vi "AuMT8852B EDR Relative Transmit Power Results.vi"(8 "error in (no error)":errorcluster, 11 "VISA session":refnum<visa-resource-name>) -> (0 "error out":errorcluster, 2 "error code":i32, 3 "VISA session out":refnum<visa-resource-name>, 4 "Results":T1 {"Peak 2DHx DPSK Absolute Power (dBm)" format="%.2f"; "Avg 2DHx DPSK Absolute Power (dBm)" format="%.2f"; "Min 2DHx DPSK Absolute Power (dBm)" format="%.2f"; "Max 2DHx DPSK Absolute Power (dBm)" format="%.2f"; "Peak 2DHx GFSK Absolute Power (dBm)" format="%.2f"; "Avg 2DHx GFSK Absolute Power (dBm)" format="%.2f"; "Min 2DHx GFSK Absolute Power (dBm)" format="%.2f"; "Max 2DHx GFSK Absolute Power (dBm)" format="%.2f"; "Peak 3DHx DPSK Absolute Power (dBm)" format="%.2f"; "Avg 3DHx DPSK Absolute Power (dBm)" format="%.2f"; "Min 3DHx DPSK Absolute Power (dBm)" format="%.2f"; "Max 3DHx DPSK Absolute Power (dBm)" format="%.2f"; "Peak 3DHx GFSK Absolute Power (dBm)" format="%.2f"; "Avg 3DHx GFSK Absolute Power (dBm)" format="%.2f"; "Min 3DHx GFSK Absolute Power (dBm)" format="%.2f"; "Max 3DHx GFSK Absolute Power (dBm)" format="%.2f"; "Avg power difference (dBm)" format="%.2f"; "Min power difference (dBm)" format="%.2f"; "Max power difference (dBm)" format="%.2f"; "Avg power difference (dBm)" format="%.2f"; "Min power difference (dBm)" format="%.2f"; "Max power difference (dBm)" format="%.2f"})   [LabVIEW 2017]
doc: "Anritsu MT8852B Bluetooth Tester\n\nReturns the summary results of the EDR Relative Transmit Power test.\n\nOUTPUT\nResults - measurements made during the test."
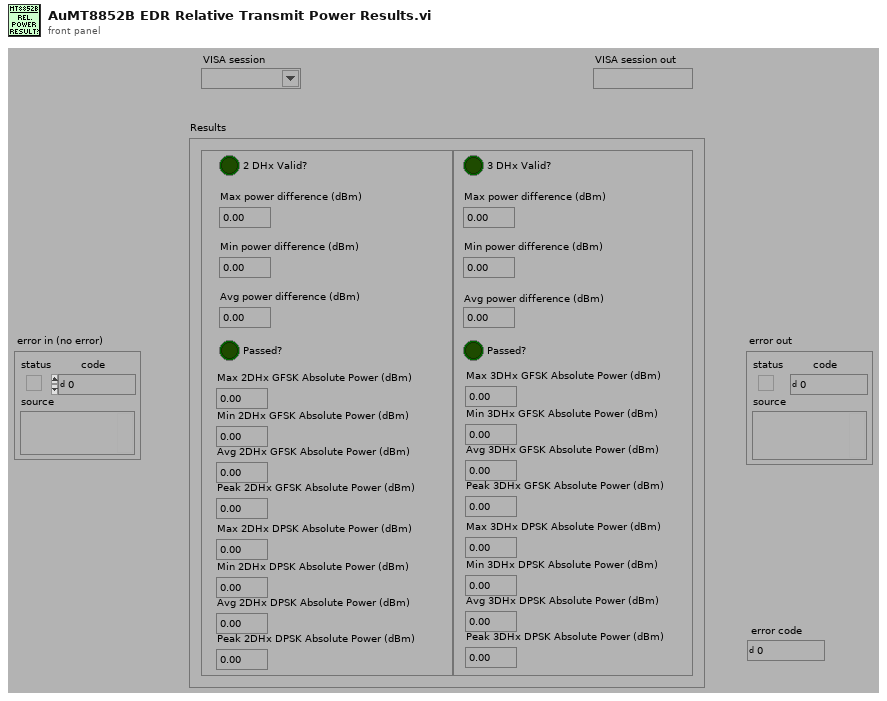
[diagram p1: front panel]
types:
  T1 = cluster{"2 DHx Valid?":bool, "Max power difference (dBm)":dbl, "Min power difference (dBm)":dbl, "Avg power difference (dBm)":dbl, "Passed?":bool, "3 DHx Valid?":bool, "Max power difference (dBm)":dbl, "Min power difference (dBm)":dbl, "Avg power difference (dBm)":dbl, "Passed?":bool, "Max 3DHx GFSK Absolute Power (dBm)":dbl, "Min 3DHx GFSK Absolute Power (dBm)":dbl, "Avg 3DHx GFSK Absolute Power (dBm)":dbl, "Peak 3DHx GFSK Absolute Power (dBm)":dbl, "Max 3DHx DPSK Absolute Power (dBm)":dbl, "Min 3DHx DPSK Absolute Power (dBm)":dbl, "Avg 3DHx DPSK Absolute Power (dBm)":dbl, "Peak 3DHx DPSK Absolute Power (dBm)":dbl, "Max 2DHx GFSK Absolute Power (dBm)":dbl, "Min 2DHx GFSK Absolute Power (dBm)":dbl, "Avg 2DHx GFSK Absolute Power (dBm)":dbl, "Peak 2DHx GFSK Absolute Power (dBm)":dbl, "Max 2DHx DPSK Absolute Power (dBm)":dbl, "Min 2DHx DPSK Absolute Power (dBm)":dbl, "Avg 2DHx DPSK Absolute Power (dBm)":dbl, "Peak 2DHx DPSK Absolute Power (dBm)":dbl}
  T2 = enum16{"Simulate", "Range check", "Cache", "Query instrument status"}
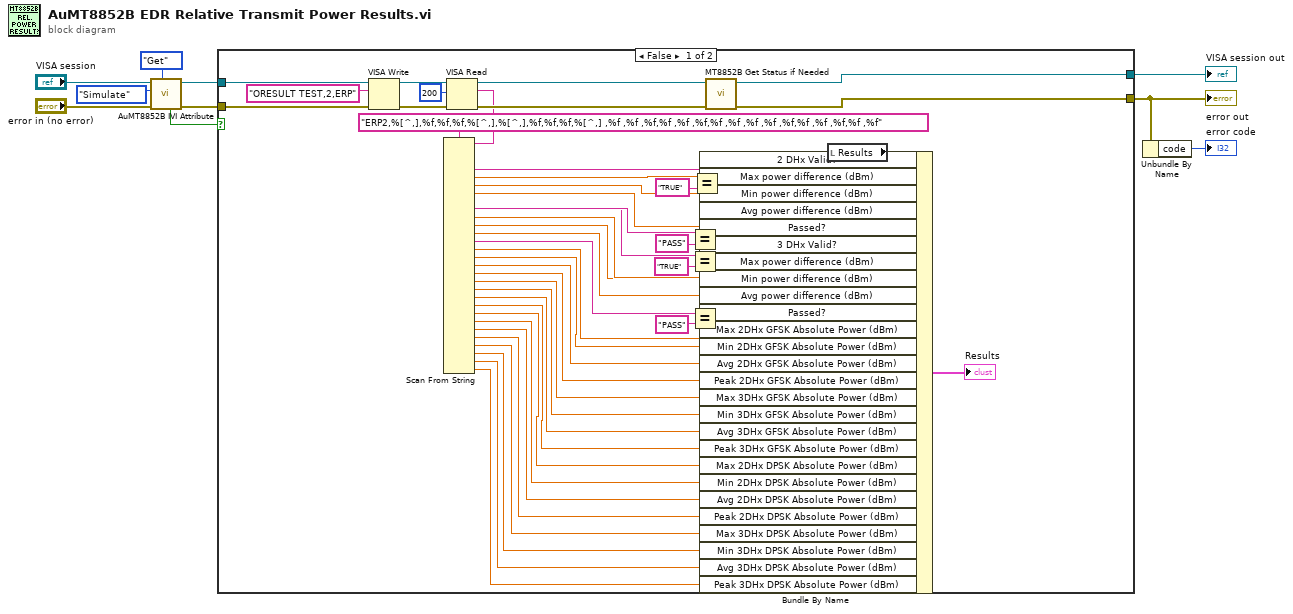
[diagram p0: block diagram]
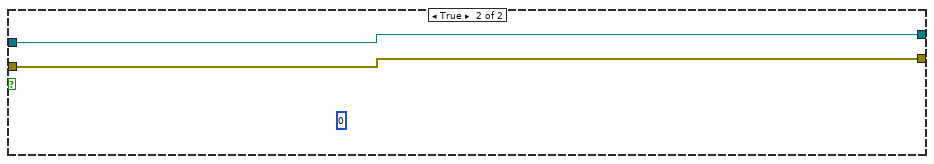
[diagram p2: hidden frame]
diagram:
  n1 = call <instrlib>:"AuMT8852B IVI Attribute.vi"("Set/Get (Set)"=enum16{"Set", "Get"}."Get", "error in (no error)"="error in (no error)", "Flag (Simulate)"=T2."Simulate", "VISA session"="VISA session") -> ("error out"=w7:errorcluster, "VISA session out"=w9:refnum<visa-resource-name>, "Value out"=w3:bool)  [unwired: 5 in]
  n2 = case shown="False" w3 {
    tunnel: [w49 w60] -> w10
    tunnel: [w48 w59] -> w1
    tunnel: w9 -> [w57 w60]
    tunnel: w7 -> [w56 w59]
    frame False {
      n3 = VISA Write(VISA resource name=w57, write buffer="ORESULT TEST,2,ERP" ("write buffer (\"\")"), error in (no error)=w56) -> (VISA resource name out=w55:refnum<visa-resource-name>, error out=w54:errorcluster)  [unwired: 1 out]
      n4 = VISA Read(VISA resource name=w55, byte count=u32 200 ("byte count (0)"), error in (no error)=w54) -> (VISA resource name out=w47:refnum<visa-resource-name>, read buffer=w45:string, error out=w46:errorcluster)  [unwired: 1 out]
      n5 = Scan From String(format string="ERP2,%[^,],%f,%f,%f,%[^,],%[^,],%f,%f,%f,%[^,] ,%f ,%f ,%f,%f ,%f ,%f,%f ,%f ,%f ,%f ,%f,%f ,%f ,%f,%f ,%f" ("Format String"), input string=w45) -> (output 1=w44:string, output 2=w38:dbl, output 3=w37:dbl, output 4=w36:dbl, output 5=w40:string, output 6=w34:string, output 7=w32:dbl, output 8=w27:dbl, output 9=w31:dbl, output 10=w28:string, output 11=w26:dbl, output 12=w25:dbl, output 13=w24:dbl, output 14=w23:dbl, output 15=w22:dbl, output 16=w21:dbl, output 17=w20:dbl, output 18=w19:dbl, output 19=w18:dbl, output 20=w17:dbl, output 21=w16:dbl, output 22=w15:dbl, output 23=w14:dbl, output 24=w13:dbl, output 25=w12:dbl, output 26=w11:dbl)  [unwired: 28 in, 3 out]
      n6 = Equal?(x=w40, y="PASS") -> (x = y?=w39:bool)
      n7 = Equal?(x=w34, y="TRUE") -> (x = y?=w35:bool)
      n8 = Equal?(x=w28, y="PASS") -> (x = y?=w30:bool)
      n9 = Equal?(x=w44, y="TRUE") -> (x = y?=w41:bool)
      n10 = call <instrlib>:"MT8852B Get Status if Needed.vi"("error in (no error)"=w46, "VISA session"=w47) -> ("error out"=w48:errorcluster, "VISA session out"=w49:refnum<visa-resource-name>)  [unwired: 8 in]
      n11 = local read "Results"() -> (w42:T1)
      n12 = Bundle By Name(cluster=w42, "2 DHx Valid?"=w41, "Max power difference (dBm)"=w38, "Min power difference (dBm)"=w37, "Avg power difference (dBm)"=w36, "Passed?"=w39, "3 DHx Valid?"=w35, "Max power difference (dBm)"=w32, "Min power difference (dBm)"=w27, "Avg power difference (dBm)"=w31, "Passed?"=w30, "Max 2DHx GFSK Absolute Power (dBm)"=w26, "Min 2DHx GFSK Absolute Power (dBm)"=w25, "Avg 2DHx GFSK Absolute Power (dBm)"=w24, "Peak 2DHx GFSK Absolute Power (dBm)"=w23, "Max 3DHx GFSK Absolute Power (dBm)"=w22, "Min 3DHx GFSK Absolute Power (dBm)"=w21, "Avg 3DHx GFSK Absolute Power (dBm)"=w20, "Peak 3DHx GFSK Absolute Power (dBm)"=w19, "Max 2DHx DPSK Absolute Power (dBm)"=w18, "Min 2DHx DPSK Absolute Power (dBm)"=w17, "Avg 2DHx DPSK Absolute Power (dBm)"=w16, "Peak 2DHx DPSK Absolute Power (dBm)"=w15, "Max 3DHx DPSK Absolute Power (dBm)"=w14, "Min 3DHx DPSK Absolute Power (dBm)"=w13, "Avg 3DHx DPSK Absolute Power (dBm)"=w12, "Peak 3DHx DPSK Absolute Power (dBm)"=w11) -> (→"Results":T1)
    }
    frame True {
      (unwired) u8 0
    }
  }
  "error out" <- w1
  "VISA session out" <- w10
  n13 = Unbundle By Name(w1) -> ("code"=→"error code":i32)
